vi "MoveAbs.vi"   [LabVIEW 2018, in "Aerotech.lvlib"]
uses:
  Aerotech.lvlib
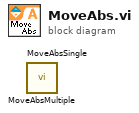
[diagram p0: block diagram]
diagram:
  n1 = call "MoveAbsMultiple.vi"() -> ()  [unwired: 10 in, 2 out]
  n2 = call "MoveAbsSingle.vi"() -> ()  [unwired: 10 in, 2 out]
